vi "Construct Configuration Object.vi"(7 "Window Title":string, 8 "error in (no error)":errorcluster, 9 "Initial Category Selection":i32=-1, 10 "Configuration File Path":path, 11 "Configuration in":refnum<class "Configuration.lvclass">) -> (0 "error out":errorcluster, 1 "Stop Event":refnum<user-event>, 2 "Path to config file":path, 3 "Configuration out":refnum<class "Configuration.lvclass">)   [LabVIEW 2016, in "Configuration.lvlib" / "Configuration.lvclass"]
uses:
  Configuration.lvclass
  <vilib>/Utility/sysdir.llb/System Directory Type.ctl
  <userlib>/_OpenG.lib/file/file.llb/File Exists - Scalar__ogtk.vi
  <userlib>/_OpenG.lib/file/file.llb/Valid Path - Traditional__ogtk.vi
  <userlib>/_OpenG.lib/file/file.llb/Convert File Extension (Path)__ogtk.vi
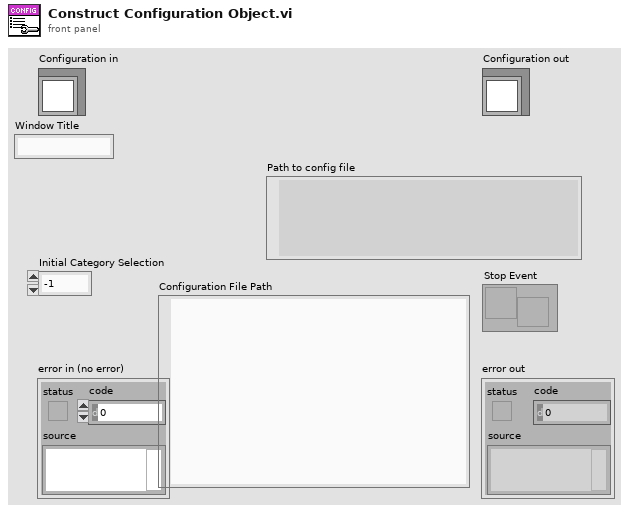
[diagram p1: front panel]
types:
  T1 = typedef "System Directory Type.ctl" = i32
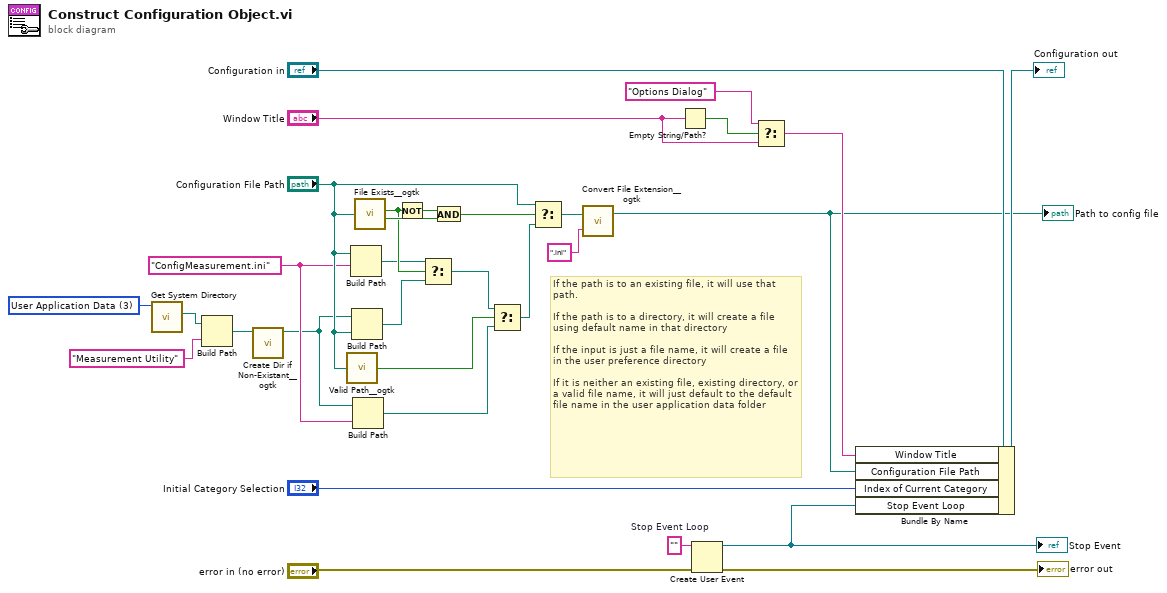
[diagram p0: block diagram]
diagram:
  w12 = "ConfigMeasurement.ini" ("name or relative path")
  w21 = T1 3 items=["User Home"=0, "User Desktop"=1, "User Documents"=2, "User Application Data"=3, "User Preferences"=4, "User Temporary"=5, "Public Documents"=6, "Public Application Data"=7, "Public Preferences"=8, "Public Cache"=13, "System Core Libraries"=9, "System Installed Libraries"=10, "Application Files"=11, "Boot Volume Root"=12] ("system directory type")
  w28 = ""  # Stop Event Loop
  # "If the path is to an existing file, it will use that path.\n\nIf the path is to a directory, it will create a file using default name in that directory\n\nIf the input is just a file name, it will create a file in the user preference directory\n\nIf it is neither an existing file, existing directory, or a valid file name, it will just default to the default file name in the user application data folder"
  n1 = call <vilib>:"Get System Directory.vi"("system directory type"=w21) -> ("system directory"=w4:path)  [unwired: 10 in]
  n2 = Build Path(base path=w4, name or relative path="Measurement Utility") -> (appended path=w2:path)
  n3 = call <userlib>:"Create Dir if Non-Existant__ogtk.vi"("Directory Path"=w2) -> ("dup Directory Path"=w1:path)  [unwired: 8 in, 2 out]
  n4 = call-poly <userlib>:"Valid Path__ogtk.vi"("path"="Configuration File Path") -> ("valid"=w11:bool)
  n5 = Build Path(base path="Configuration File Path", name or relative path=w12) -> (appended path=w15:path)
  n6 = Build Path(base path=w1, name or relative path="Configuration File Path") -> (appended path=w14:path)
  n7 = Build Path(base path=w1, name or relative path=w12) -> (appended path=w10:path)
  n8 = call-poly <userlib>:"File Exists__ogtk.vi"("file path"="Configuration File Path") -> ("is directory"=w16:bool, "exists"=w18:bool)  [unwired: 6 in]
  n9 = Not(x=w16) -> (.not. x?=w19:bool)
  n10 = Select(t=w15, s=w16, f=w14) -> (s? t:f=w9:path)
  n11 = And(x=w19, y=w18) -> (x .and. y?=w17:bool)
  n12 = Select(t=w9, s=w11, f=w10) -> (s? t:f=w8:path)
  n13 = Select(t="Configuration File Path", s=w17, f=w8) -> (s? t:f=w7:path)
  n14 = call-poly <userlib>:"Convert File Extension__ogtk.vi"("new ending (none)"=".ini" ("y"), "file name"=w7) -> ("new filename"=w5:path)  [unwired: 1 out]
  "Path to config file" <- w5
  n15 = Empty String/Path?(string/path="Window Title") -> (empty?=w25:bool)
  n16 = Create User Event(user event datatype=w28, error in="error in (no error)") -> (user event=w29:refnum<user-event>, error out=→"error out":errorcluster)
  "Stop Event" <- w29
  n17 = Select(t="Options Dialog" ("Window Title"), s=w25, f="Window Title") -> (s? t:f=w22:string)
  n18 = Bundle By Name(cluster="Configuration in", "Window Title"=w22, "Configuration File Path"=w5, "Index of Current Category"="Initial Category Selection", "Stop Event Loop"=w29) -> (→"Configuration out":refnum<class "Configuration.lvclass">)
